vi "dvotConstants.vi"() -> ()   [LabVIEW 2012]
panel:
  out "B_ALPHA":dbl=5.48e-19
  out "DENSITY_APATITE":dbl=3.19
  out "N_PER_NMOL":dbl=602214199000000.0 format="%#_9g"
  out "N_PER_MOL":dbl=6.02214199e+23 format="%#_9g"
  out "U238U235RATIO":dbl=137.88
  out "PPM_NMPG_SM147":dbl=6.80272
  out "PPM_NMPG_TH232":dbl=4.31034
  out "PPM_NMPG_U235":dbl=4.25532
  out "PPM_NMPG_U238":dbl=4.20168
  out "U238YR_SF":dbl=8.46e-17
  out "SM147SEC":dbl=2.072e-19
  out "SM147MA":dbl=6.54e-06
  out "SM147YR":dbl=6.54e-12
  out "TH232SEC":dbl=1.56781e-18
  out "TH232MA":dbl=4.9475e-05
  out "TH232YR":dbl=4.9475e-11
  out "U235SEC":dbl=3.12089e-17
  out "U235YR":dbl=9.8485e-10
  out "U235MA":dbl=0.00098485
  out "U238SEC":dbl=4.91575e-18
  out "U238MA":dbl=0.000155125
  out "U238YR":dbl=1.55125e-10 format="%#_12g"
  out "UNIV_GAS_CONST":dbl=1.987
  out "KELVINS_AT_0C":dbl=273.15
  out "SECS_PER_YR":dbl=31556925.9747 format="%#_13e"
  out "SECS_PER_MA":dbl=31556925974700.0 format="%#_13g"
  # "Fission decay constant"
  # "in g/cm3"
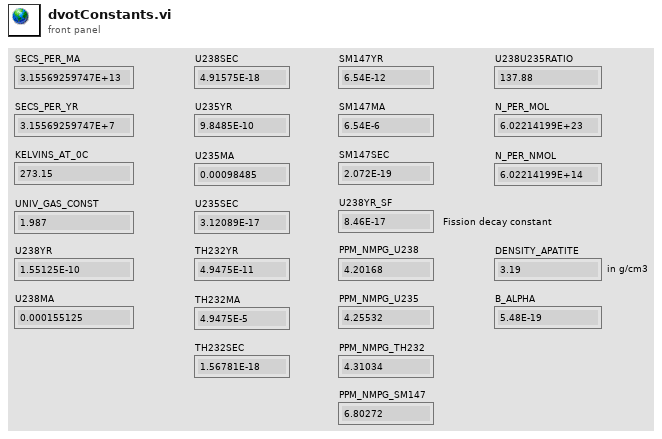
[diagram p1: front panel]
diagram:
